vi "GetLeftSideInformation.vi"(8 "error in (no error)":errorcluster, 10 "FirstCharInfo":T1, 11 "EAN in":refnum<class "EAN-13.lvclass">) -> (0 "error out":errorcluster, 2 "Text Position":T1, 3 "EAN out":refnum<class "EAN-13.lvclass">)   [LabVIEW 2013, in "BarCodes.lvlib" / "EAN-13.lvclass"]
uses:
  EAN-13.lvclass
  BarCode/TextPosition.ctl
  BarCodes.lvlib
  BarCode/BarCode.lvclass
panel:
  in  "Input":string
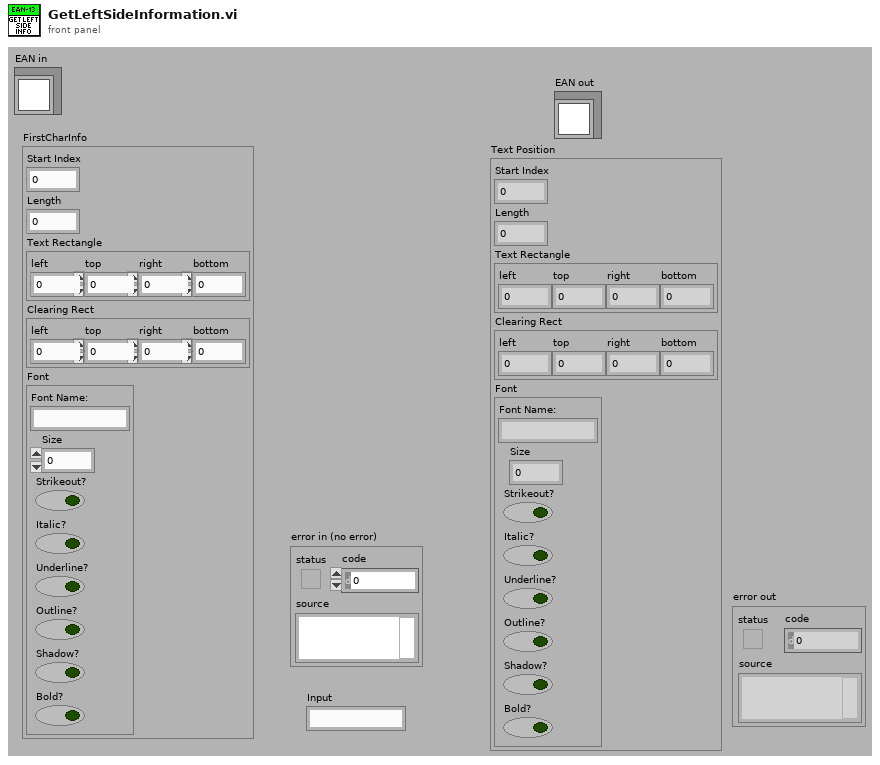
[diagram p1: front panel]
types:
  T1 = typedef "BarCodes.lvlib/BarCode.lvclass/TextPosition.ctl" = cluster{"Start Index":u8, "Length":u8, "Text Rectangle":cluster{"left":i16, "top":i16, "right":i16, "bottom":i16}, "Clearing Rect":cluster{"left":i16, "top":i16, "right":i16, "bottom":i16}, "Font":cluster{"Font Name:":string, "Size":i16, "Strikeout?":bool, "Italic?":bool, "Underline?":bool, "Outline?":bool, "Shadow?":bool, "Bold?":bool}}
  T2 = cluster{"left":i32, "top":i16, "right":i16, "bottom":i16}
  T3 = cluster{"left":i16, "top":i16, "right":i16, "bottom":i16}
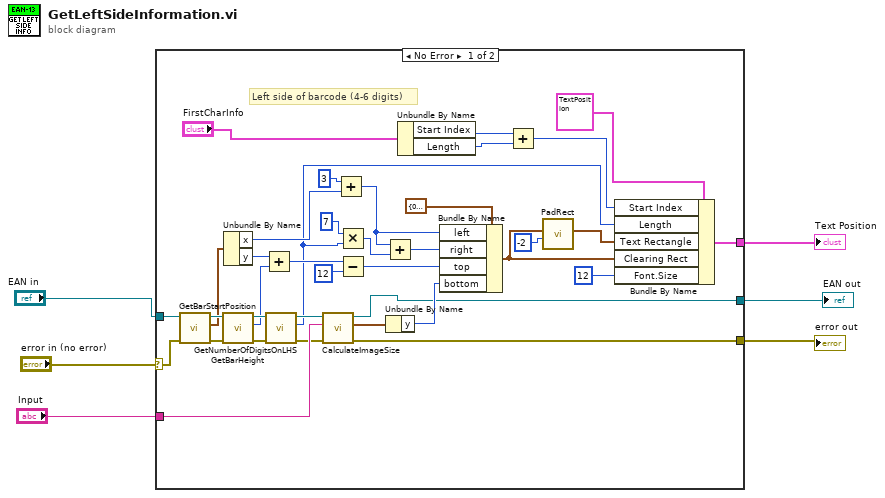
[diagram p0: block diagram]
diagram:
  n1 = case shown="No Error" "error in (no error)" {
    selector: "error in (no error)" -> [w13 w45]
    tunnel: "Input" -> [w42 _]
    tunnel: [w40 _] -> w5
    tunnel: "EAN in" -> [w37 w44]
    tunnel: [w14 w45] -> w3
    tunnel: [w12 w44] -> w1
    frame No Error {
      # "Left side of barcode (4-6 digits)"
      n2 = call-dynamic "GetBarStartPosition.vi"("error in (no error)"=w13, "EAN-13 in"=w37) -> ("error out"=w17:errorcluster, "Start Position"=w35:cluster{"x":i16, "y":i16}, "EAN-13 out"=w36:refnum<class "EAN-13.lvclass">)  [unwired: 7 in]
      n3 = call-dynamic "GetBarHeight.vi"("error in (no error)"=w17, "EAN-13 in"=w36) -> ("error out"=w16:errorcluster, "Bar Height"=w38:u8, "EAN-13 out"=w39:refnum<class "EAN-13.lvclass">)  [unwired: 7 in]
      n4 = Unbundle By Name(w35) -> ("x"=w34:i16, "y"=w33:i16)
      n5 = Add(x=w33, y=w38) -> (x+y=w20:i16)
      n6 = call-dynamic "GetNumberOfDigitsOnLHS.vi"("error in (no error)"=w16, "EAN-13 in"=w39) -> ("error out"=w15:errorcluster, "NumberOfDigitsOnLHS"=w11:u8, "EAN-13 out"=w18:refnum<class "EAN-13.lvclass">)  [unwired: 7 in]
      n7 = call-dynamic "CalculateImageSize.vi"("error in (no error)"=w15, "String"=w42, "EAN-13 in"=w18) -> ("error out"=w14:errorcluster, "Size"=w24:cluster{"x":i16, "y":i16}, "EAN-13 out"=w12:refnum<class "EAN-13.lvclass">)  [unwired: 6 in]
      n8 = Add(x=i16 3, y=w34) -> (x+y=w29:i16)
      n9 = Multiply(x=u8 7, y=w11) -> (x*y=w28:u8)
      n10 = Subtract(x=w20, y=i16 12 ("x")) -> (x-y=w25:i16)
      n11 = Add(x=w29, y=w28) -> (x+y=w27:i16)
      n12 = Unbundle By Name(w24) -> ("y"=w23:i16)
      n13 = Unbundle By Name("FirstCharInfo") -> ("Start Index"=w9:u8, "Length"=w8:u8)
      n14 = Bundle By Name(cluster=T2 {"left"=0, "top"=0, "right"=0, "bottom"=0} ("Text Rectagle"), "left"=w29, "right"=w27, "top"=w25, "bottom"=w23) -> (w21:T2)
      n15 = Add(x=w9, y=w8) -> (x+y=w7:u8)
      n16 = call "PadRect.vi"("Padding"=i8 -2, "Rectagle"=w21) -> ("Padded Rectangle"=w22:T3)  [unwired: 9 in]
      n17 = Bundle By Name(cluster=T1 {"Start Index"=0, "Length"=0, "Text Rectangle"={"left"=0, "top"=0, "right"=0, "bottom"=0}, "Clearing Rect"={"left"=0, "top"=0, "right"=0, "bottom"=0}, "Font"={"Font Name:"="Application Font", "Size"=12, "Strikeout?"=FALSE, "Italic?"=FALSE, "Underline?"=FALSE, "Outline?"=FALSE, "Shadow?"=FALSE, "Bold?"=FALSE}} ("Text Position"), "Start Index"=w7, "Length"=w11, "Text Rectangle"=w22, "Clearing Rect"=w21, "Font.Size"=i16 12) -> (w40:T1)
    }
    frame Error {
    }
  }
  "Text Position" <- w5
  "error out" <- w3
  "EAN out" <- w1
